vi "External Sensor Offsets Dataset.vi"(7 "Number of Sensors":i32, 8 "error in (no error)":errorcluster, 10 "Offsets In":dbl[](array[numeric]), 11 "DAO Actions":T1) -> (0 "error out":errorcluster, 2 "Offsets Out":dbl[](array[numeric]))   [LabVIEW 2009]
uses:
  Data Access Objects/Metadata/DAO Actions.ctl
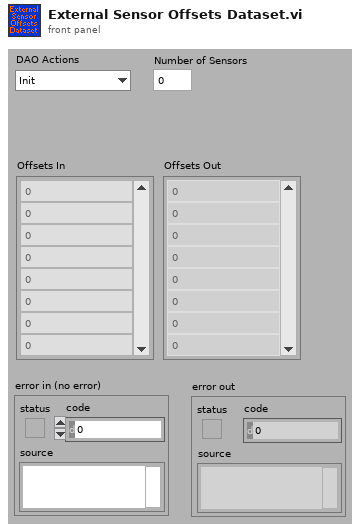
[diagram p1: front panel]
types:
  T1 = typedef "DAO Actions.ctl" = enum16{"Init", "Get", "Set"}
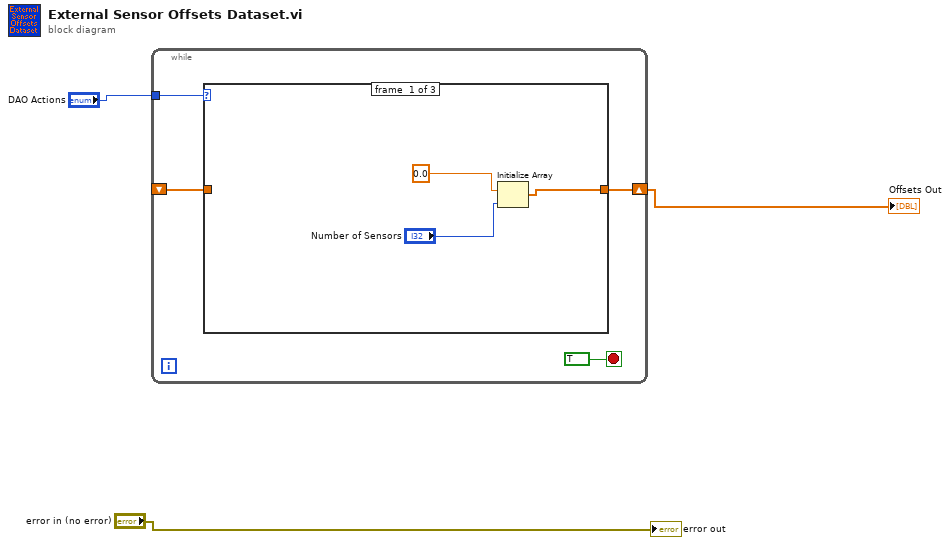
[diagram p0: block diagram]
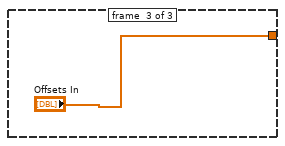
[diagram p3: hidden frame]
diagram:
  n1 = while {
    tunnel: "DAO Actions" -> [w6]
    shift-right: [w5] -> w1
    shift-left: _ -> [w4]
    stop <- TRUE stop-if-true
    n2 = case shown="\"Set\"" w6 {
      tunnel: [w8 w11 "Offsets In"] -> w5
      tunnel: w4 -> [_ w11 _]
      frame #0 {
        n3 = Initialize Array(0.0, "Number of Sensors") -> (w8:dbl[])
      }
      frame #1 {
      }
      frame #2 {
      }
    }
  }
  "Offsets Out" <- w1
  "error out" <- "error in (no error)"
